vi "frequencies.vi"(8 "Error in":errorcluster, 11 "VISA name in":refnum<visa-resource-name>) -> (0 "Error out":errorcluster, 2 "Frequency (Hz)":dbl[](array[numeric]), 3 "VISA name out":refnum<visa-resource-name>)   [LabVIEW 2012]
panel:
  out "cmd echo":string="\r\n"
  out "i":i32
  out "response":string
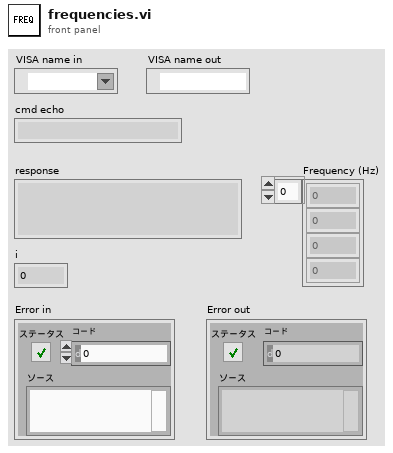
[diagram p1: front panel]
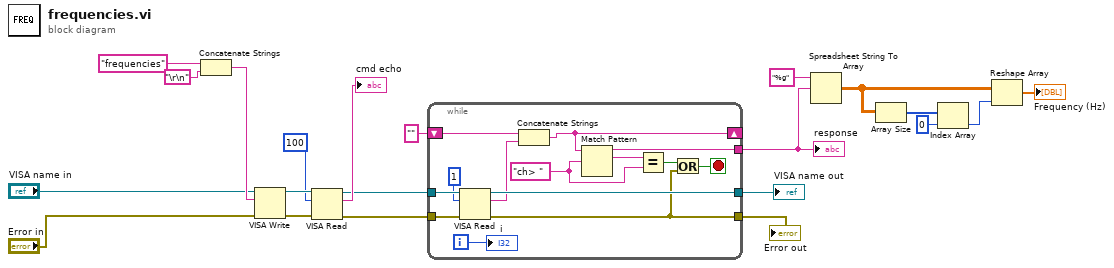
[diagram p0: block diagram]
diagram:
  n1 = Concatenate Strings("frequencies" ("形式文字列"), "\r\n") -> (w20:string)
  n2 = VISA Write(VISA resource name="VISA name in", write buffer=w20, error in (no error)="Error in") -> (VISA resource name out=w17:refnum<visa-resource-name>, error out=w16:errorcluster)  [unwired: 1 out]
  n3 = VISA Read(VISA resource name=w17, byte count=u32 100 ("バイトカウント"), error in (no error)=w16) -> (VISA resource name out=w13:refnum<visa-resource-name>, read buffer=→"cmd echo":string, error out=w12:errorcluster)  [unwired: 1 out]
  n4 = while {
    shift-right: [w29] -> _
    shift-left: "" -> [w30]
    tunnel: [w28] -> w7
    tunnel: w13 -> [w35]
    tunnel: [w32] -> w10
    tunnel: w12 -> [w34]
    tunnel: [w22] -> w9
    i -> [w25]
    stop <- w24 stop-if-true
    w26 = "ch> " ("正規表現")
    n5 = VISA Read(VISA resource name=w35, byte count=u32 1 ("バイトカウント"), error in (no error)=w34) -> (VISA resource name out=w32:refnum<visa-resource-name>, read buffer=w31:string, error out=w22:errorcluster)  [unwired: 1 out]
    n6 = Concatenate Strings(w30, w31) -> (w29:string)
    n7 = Match Pattern(string=w29, regular expression=w26) -> (before substring=w28:string, match substring=w27:string)  [unwired: 1 in, 2 out]
    n8 = Equal?(x=w27, y=w26) -> (x = y?=w23:bool)
    n9 = Or(x=w23, y=w22) -> (x .or. y?=w24:bool)
    "i" <- w25
  }
  "response" <- w7
  "VISA name out" <- w10
  "Error out" <- w9
  n10 = Spreadsheet String To Array(format string="%g" ("形式文字列"), spreadsheet string=w7) -> (array=w3:dbl[][])  [unwired: 2 in]
  n11 = Array Size(array=w3) -> (size(s)=w5:i32[])
  n12 = Index Array(array=w5, index=0 ("指標")) -> (element=w2:i32)
  n13 = Reshape Array(w3, w2) -> (→"Frequency (Hz)":dbl[])
